vi "Get settings chain.vi"(8 "error in (no error)":errorcluster, 11 "ServiceManager in":refnum<class "ServiceManager.lvclass">) -> (0 "error out":errorcluster, 1 "class name":string[](array[string]), 2 "settings":variant[](array[variant]), 3 "ServiceManager out":refnum<class "ServiceManager.lvclass">)   [LabVIEW 2012, in "ServiceManager.lvclass"]
doc: "Returns an array of variants containing the settings clusters of each class in the inheritance chain (lowest child class first), together with an array of all class names in the inheritance chain.\n\nFor classes without settings cluster, the settings chain contains empty variants."
uses:
  ServiceManager.lvclass
  <vilib>/Distrio/Murmex/Murmex/Murmex.lvclass
  ServiceManager.lvclass/ServiceManager.ctl
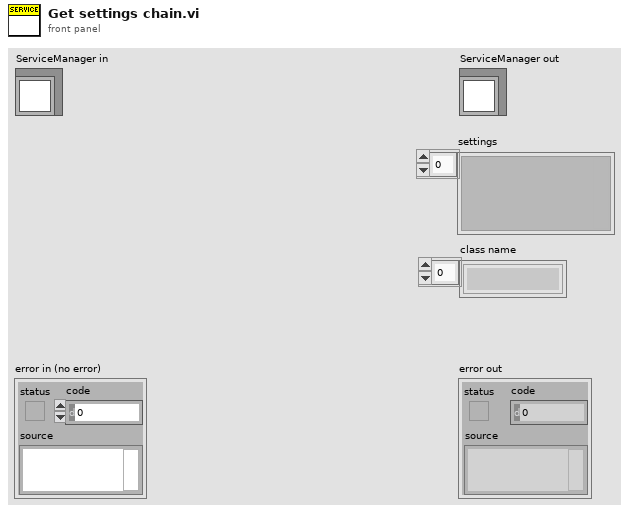
[diagram p1: front panel]
types:
  T1 = typedef "ServiceManager.lvclass/settings_cluster.ctl" = cluster{"components":T2[]}
  T2 = typedef "Murmex.lvlib/Murmex.lvclass/component_specification_cluster.ctl" = cluster{"name":string, "language":string, "host name":string, "id":string}
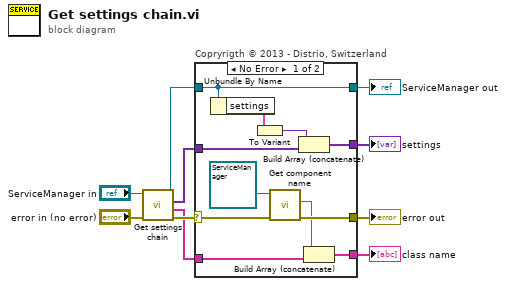
[diagram p0: block diagram]
diagram:
  n1 = call-parent "Get settings chain.vi"("error in (no error)"="error in (no error)", "MurmexBase in"="ServiceManager in") -> ("error out"=w8:errorcluster, "class name"=w6:string[], "settings"=w5:variant[], "MurmexBase out"=w7:refnum<class "ServiceManager.lvclass">)  [unwired: 6 in]
  n2 = case "Copryrigth © 2013 - Distrio, Switzerland" shown="No Error" w8 {
    selector: w8 -> [w21 w23]
    tunnel: [w20 w23] -> w3
    tunnel: [w11 w22] -> w4
    tunnel: w7 -> [w11 w22]
    tunnel: [w18 _] -> w2
    tunnel: [w17 _] -> w1
    tunnel: w6 -> [w16 _]
    tunnel: w5 -> [w15 _]
    frame No Error {
      n3 = Unbundle By Name(w11) -> ("settings"=w14:T1)
      n4 = To Variant(anything=w14) -> (Variant=w13:variant)
      n5 = call <vilib>:"Get component name.vi"("error in (no error)"=w21, "Murmex in"=refnum<class "ServiceManager.lvclass"> refnum ("ServiceManager in")) -> ("error out"=w20:errorcluster, "component name"=w19:string)  [unwired: 7 in, 1 out]
      n6 = Build Array (concatenate)(w13, w15) -> (w17:variant[])
      n7 = Build Array (concatenate)(w19, w16) -> (w18:string[])
    }
    frame Error {
    }
  }
  "error out" <- w3
  "ServiceManager out" <- w4
  "settings" <- w1
  "class name" <- w2
